vi "SetSRCreationDateEnd(SubVI).vi"(10 "seconds since 1Jan1904":timestamp, 11 "HTTP string in":string) -> (3 "String":string)   [LabVIEW 2018, in "Controller.lvlib"]
uses:
  Controller.lvlib
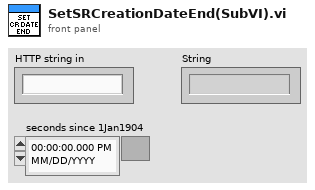
[diagram p1: front panel]
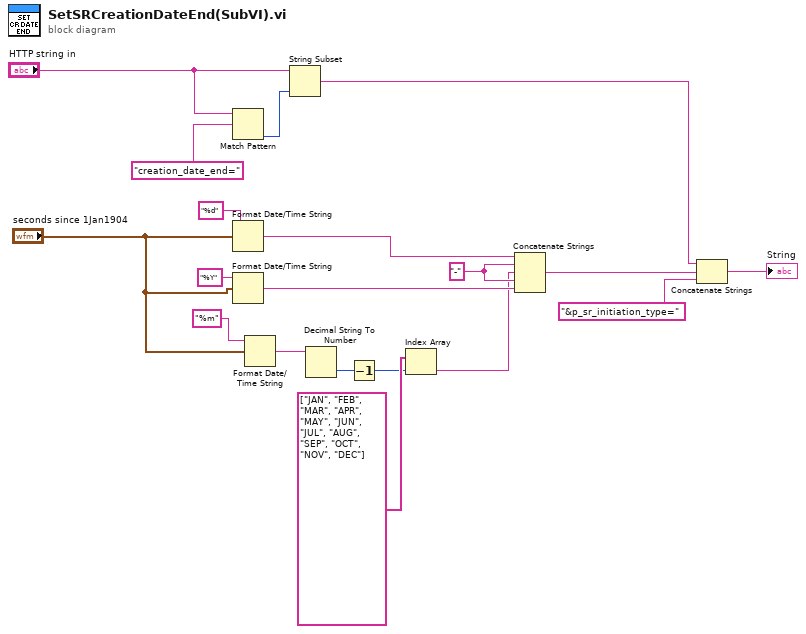
[diagram p0: block diagram]
diagram:
  w15 = "-" ("string")
  n1 = Match Pattern(string="HTTP string in", regular expression="creation_date_end=") -> (offset past match=w10:i32)  [unwired: 1 in, 3 out]
  n2 = Format Date/Time String(time format string (%c)="%d", seconds (now)="seconds since 1Jan1904") -> (date/time string=w14:string)  [unwired: 1 in]
  n3 = Format Date/Time String(time format string (%c)="%Y", seconds (now)="seconds since 1Jan1904") -> (date/time string=w16:string)  [unwired: 1 in]
  n4 = Format Date/Time String(time format string (%c)="%m", seconds (now)="seconds since 1Jan1904") -> (date/time string=w6:string)  [unwired: 1 in]
  n5 = String Subset(string="HTTP string in", length (rest)=w10) -> (substring=w8:string)  [unwired: 1 in]
  n6 = Decimal String To Number(string=w6) -> (number=w2:i32)  [unwired: 2 in, 1 out]
  n7 = Decrement(x=w2) -> (x-1=w1:i32)
  n8 = Index Array(array=string[] ["JAN", "FEB", "MAR", "APR", "MAY", "JUN", "JUL", "AUG", "SEP", "OCT", "NOV", "DEC"], index=w1) -> (element=w3:string)
  n9 = Concatenate Strings(w14, w15, w3, w15, w16) -> (w19:string)
  n10 = Concatenate Strings(w8, w19, "&p_sr_initiation_type=" ("string")) -> (→"String":string)
